vi "Convert Alarm Status.vi"(8 "error in (no error)":errorcluster, 9 "Alarm Status String (\"\")":string, 11 "VISA resource name":refnum<visa-resource-name>) -> (0 "error out":errorcluster, 1 "Alarm Level":i32(ring) items=["No Alarm", "High Limit Alarm (H)", "Low Limit Alarm (L)", "Difference High Limit Alarm (h)", "Difference Low Limit Alarm (l)", "High Limit on Rate-of-change Alarm (R)", "Low Limit on Rate-of-change Alarm (r)", "Delay High Limit Alarm (T)", "Delay Low Limit Alarm (t)"], 3 "VISA resource name out":refnum<visa-resource-name>)   [LabVIEW 2020, in "Yokogawa GX Series.lvlib"]
doc: "This VI converts 1 character to a value as alarm status."
uses:
  <instrlib>/Yokogawa GX Series/Yokogawa GX Series.lvlib
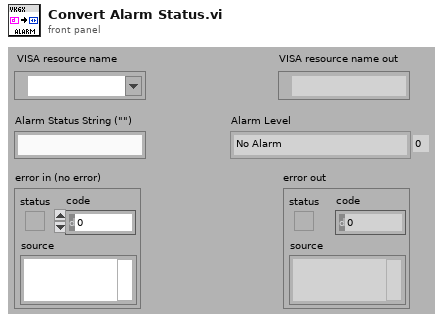
[diagram p1: front panel]
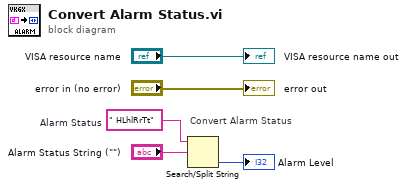
[diagram p0: block diagram]
diagram:
  w2 = " HLhlRrTt"  # Alarm Status
  # "Convert Alarm Status"
  n1 = Search/Split String(string=w2, search string/char (-)="Alarm Status String (\"\")") -> (offset of match=→"Alarm Level":i32)  [unwired: 3 out]
  "VISA resource name out" <- "VISA resource name"
  "error out" <- "error in (no error)"
